vi "FPGA.vi"() -> ()   [LabVIEW 2015]
uses:
  States.ctl
  <vilib>/rvi/Emulation/niFpgaGetClockAttributes.vi
  <vilib>/rvi/Emulation/niFpgaSctlEmulationGetInTimedLoop.vi
  <vilib>/rvi/Emulation/niFpgaEmulationReportErrorSimple.vi
  <vilib>/rvi/eio/common/nirviEmuTemplateMethod_errors.vi
  <vilib>/rvi/Emulation/niFpgaCriticalErrorInLSC.vi
  <vilib>/eio/EIONode/EIONode.xnode
panel:
  in  "Pause":u8
  in  "SPI":T1(ring)
  in  "Delay":u16
  in  "Write":bool
  out "PIC Monitor":u32
  in  "Data":u32
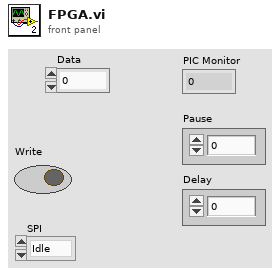
[diagram p1: front panel]
types:
  T1 = enum16{"Idle", "While loop", "Set PIC", "Bits16"}
  T2 = typedef "States.ctl" = enum16{"Idle", "CS", "Ready", "Clock High", "Clock Low", "Wait", "Exit"}
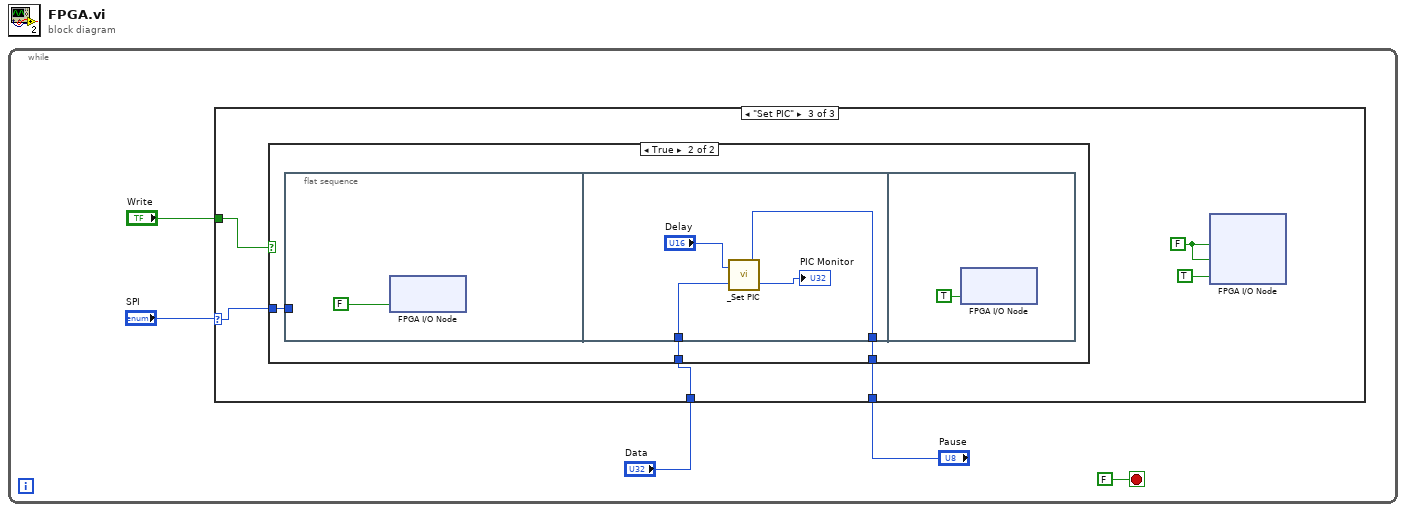
[diagram p0: block diagram]
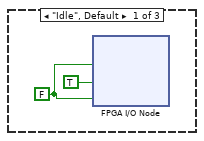
[diagram p2: hidden frame]
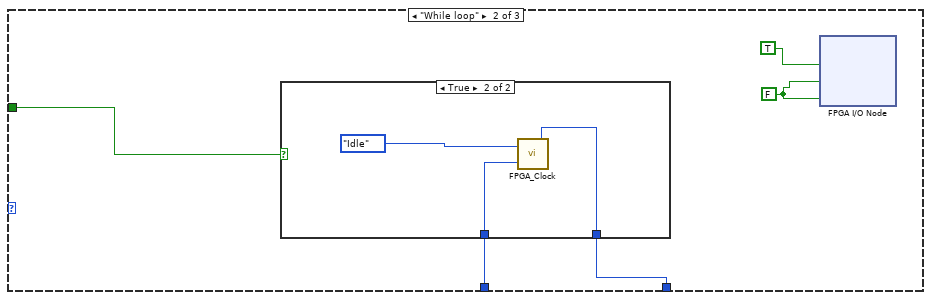
[diagram p3: hidden frame]
diagram:
  n1 = while {
    stop <- FALSE stop-if-true
    n2 = case shown="\"Set PIC\"" "SPI" {
      selector: "SPI" -> [_ _ w21]
      tunnel: "Data" -> [_ w12 w20]
      tunnel: "Write" -> [_ w11 w19]
      tunnel: "Pause" -> [_ w8 w16]
      frame "Idle", Default {
        w7 = FALSE
        n3 = xnode "FPGA I/O Node"("LED 1"=w7, "LED 2"=TRUE, "LED 3"=w7) -> ()  [unwired: 3 in, 3 out]
      }
      frame "While loop" {
        w10 = FALSE
        n4 = case shown="True" w11 {
          tunnel: w12 -> [_ w15]
          tunnel: w8 -> [_ w13]
          frame False {
          }
          frame True {
            n5 = call "FPGA_Clock.vi"("Pause"=w13, "Data"=w15, "State"=States."Idle") -> ()
          }
        }
        n6 = xnode "FPGA I/O Node"("LED 1"=TRUE, "LED 2"=w10, "LED 3"=w10) -> ()  [unwired: 3 in, 3 out]
      }
      frame "Set PIC" {
        w17 = FALSE ("CS")
        n7 = case shown="True" w19 {
          tunnel: w21 -> [_ w24]
          tunnel: w20 -> [_ w23]
          tunnel: w16 -> [_ w22]
          frame False {
          }
          frame True {
            n8 = flat-sequence {
              tunnel: w24 -> [_]
              tunnel: w23 -> [w27]
              tunnel: w22 -> [w26]
              frame #0 {
                n9 = xnode "FPGA I/O Node"("CS"=FALSE) -> ()  [unwired: 1 in, 1 out]
              }
              frame #1 {
                n10 = call "_Set PIC.vi"("Count(uSec)"=w26, "Data"=w27, "Delay"="Delay") -> ("PIC Monitor"=→"PIC Monitor":u32)
              }
              frame #2 {
                n11 = xnode "FPGA I/O Node"("CS"=TRUE) -> ()  [unwired: 1 in, 1 out]
              }
            }
          }
        }
        n12 = xnode "FPGA I/O Node"("LED 1"=w17, "LED 2"=w17, "LED 3"=TRUE ("CS")) -> ()  [unwired: 3 in, 3 out]
      }
    }
  }
